vi "Build Control Type.vi"(8 "error in (no error)":errorcluster, 11 "Button Builder.lvclass":refnum<class "Button_Builder.lvclass">) -> (0 "error out":errorcluster, 2 "GUI Control":refnum<class "GUI Control.lvclass">, 3 "Button Builder.lvclass out":refnum<class "Button_Builder.lvclass">)   [LabVIEW 2015, in "Button_Builder.lvclass"]
uses:
  Button_Builder.lvclass
  GUI Controls/GUI Control/GUI Control.lvclass
  Panel Control/Panel Data/Type Definition/Panel Control Maker State Variable.ctl
  GUI Controls/Button_UI/Button_UI.lvclass
  Panel Control_Ref/Panel Controller.lvclass
  <vilib>/Utility/error.llb/Error Cluster From Error Code.vi
  <vilib>/ErrorRing/Error Ring.xnode
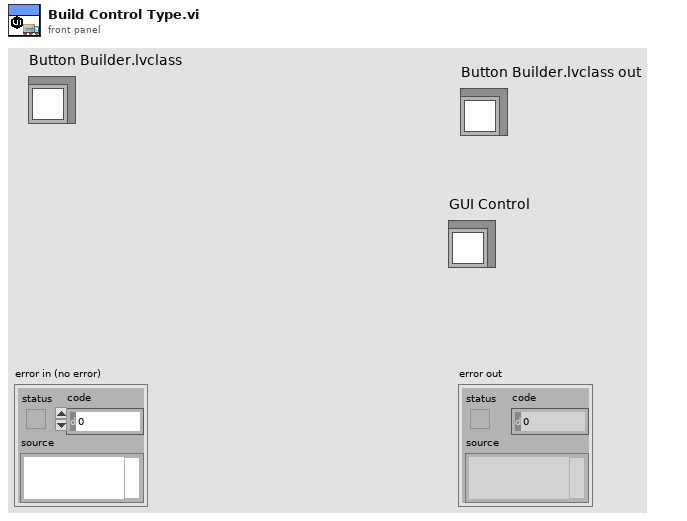
[diagram p1: front panel]
types:
  T1 = typedef "Panel Controller.lvclass/Panel Control Maker State Variable.ctl" = enum16{"Panel On", "Working", "Panel Off", "Ending"}
  T2 = enum32{"Invalid", "Standard", "Closed", "Hidden", "Minimized", "Maximized"}
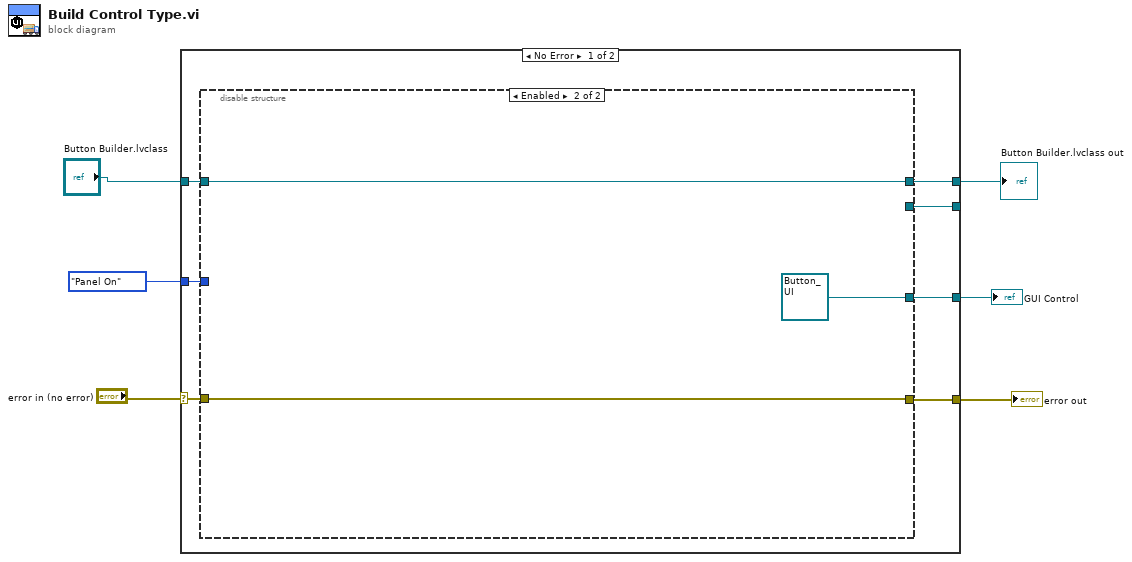
[diagram p0: block diagram]
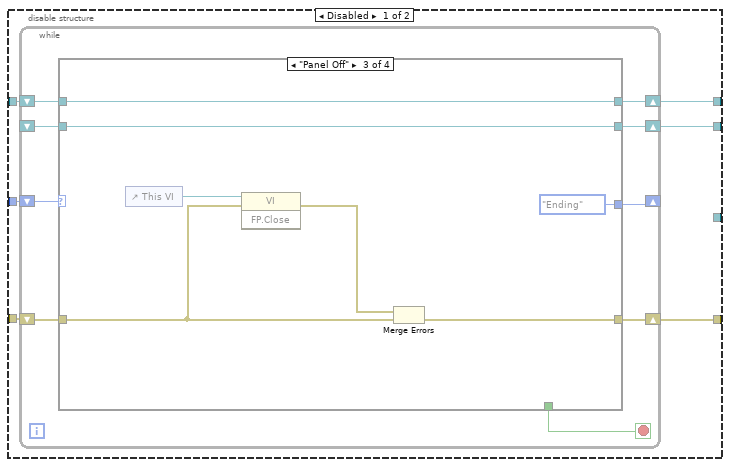
[diagram p2: hidden frame]
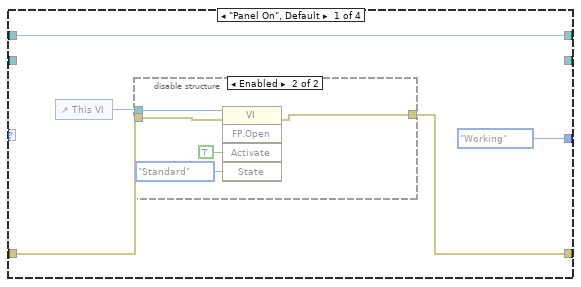
[diagram p3: hidden frame]
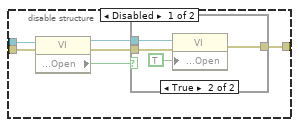
[diagram p4: hidden frame]
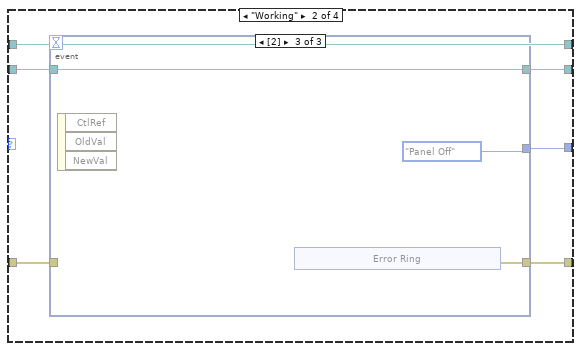
[diagram p6: hidden frame]
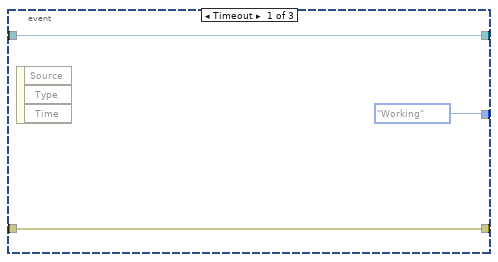
[diagram p7: hidden frame]
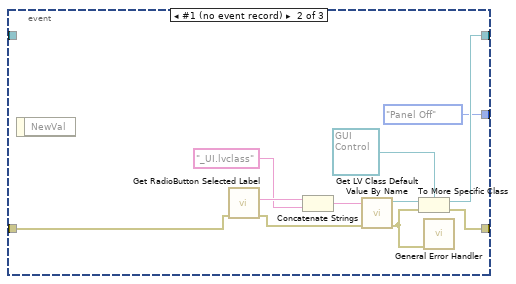
[diagram p8: hidden frame]
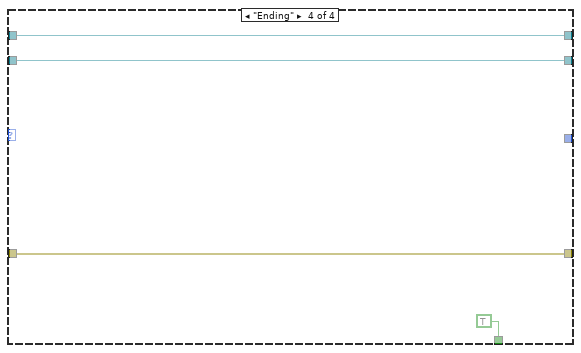
[diagram p9: hidden frame]
diagram:
  n1 = case shown="No Error" "error in (no error)" {
    selector: "error in (no error)" -> [w12 w94]
    tunnel: Panel_Control_Maker_State_Variable."Panel On" -> [w13 _]
    tunnel: [w11 w94] -> w4
    tunnel: [w10 _] -> _
    tunnel: "Button Builder.lvclass" -> [w9 w93]
    tunnel: [w8 w93] -> w1
    tunnel: [w7 _] -> w3
    frame No Error {
      n2 = disable-structure shown="Enabled" {
        disable-tunnel: w13 -> [w19 _]
        disable-tunnel: w12 -> [w18 w90]
        disable-tunnel: [w17 w90] -> w11
        disable-tunnel: [w16 _] -> w10
        disable-tunnel: w9 -> [w15 w92]
        disable-tunnel: [w14 w92] -> w8
        disable-tunnel: [_ refnum<class "Button_UI.lvclass"> refnum ("Button_UI")] -> w7
        frame Disabled {
          n3 = while {
            shift-right: [w25] -> _
            shift-left: w19 -> [w28]
            shift-right: [w26] -> w17
            shift-left: w18 -> [w27]
            shift-right: [w24] -> w16
            shift-left: _ -> [w23]
            shift-right: [w20] -> w14
            shift-left: w15 -> [w21]
            stop <- w22 stop-if-true
            n4 = case shown="\"Panel Off\"" w28 {
              tunnel: w27 -> [w32 w51 w81 w88]
              tunnel: [w31 w52 w83 w88] -> w26
              tunnel: [Panel_Control_Maker_State_Variable."Working" w53 Panel_Control_Maker_State_Variable."Ending" _] -> w25
              tunnel: [_ w55 w85 w86] -> w24
              tunnel: w23 -> [_ w54 w85 w86]
              tunnel: [_ _ _ TRUE] -> w22
              tunnel: w21 -> [w29 w50 w79 w87]
              tunnel: [w29 w50 w79 w87] -> w20
              frame "Panel On", Default {
                n5 = control-ref of="This VI"() -> (w33:refnum<vi>)
                n6 = disable-structure shown="Enabled" {
                  disable-tunnel: w33 -> [w39 w49]
                  disable-tunnel: w32 -> [w38 w48]
                  disable-tunnel: [w34 w47] -> w31
                  frame Disabled {
                    n7 = property class="VI"(reference=w39, error in=w38) -> (reference out=w35:refnum<vi>, error out=w36:errorcluster, "Front Panel.Open"=w37:bool)
                    n8 = case shown="True" w37 {
                      tunnel: w36 -> [w40 w43]
                      tunnel: w35 -> [_ w44]
                      tunnel: [w40 w41] -> w34
                      frame False {
                      }
                      frame True {
                        n9 = property class="VI"(reference=w44, error in=w43, "Front Panel.Open"=TRUE ("Front Panel Window:Open")) -> (error out=w41:errorcluster)  [unwired: 1 out]
                      }
                    }
                  }
                  frame Enabled {
                    n10 = invoke class="VI" method="FP.Open"(reference=w49, error in=w48, "Activate"=TRUE ("Activate?"), "State"=T2."Standard") -> (error out=w47:errorcluster)  [unwired: 1 in, 4 out]
                  }
                }
              }
              frame "Working" {
                n11 = event shown="[2]" {
                  selector: _ -> [_ _ _]
                  dyn-events: _ -> [_ _ _]
                  timeout: _ -> [_ _ _]
                  tunnel: [w56 w64 w73] -> w52
                  tunnel: [w57 w63 w72] -> w55
                  tunnel: w54 -> [w57 _ w72]
                  tunnel: [Panel_Control_Maker_State_Variable."Working" Panel_Control_Maker_State_Variable."Panel Off" Panel_Control_Maker_State_Variable."Panel Off"] -> w53
                  tunnel: w51 -> [w56 w61 _]
                  event Timeout {
                    n12 = event-data() -> ()  [unwired: 1 in, 3 out]
                  }
                  event #1 (no event record) {
                    n13 = event-data() -> ()  [unwired: 1 in, 1 out]
                    n14 = call "Get RadioButton Selected Label.vi"("error in (no error)"=w61) -> ("error out"=w60:errorcluster, "Label.Text"=w69:string, "Radio Buttons"=w70:refnum<vi>)  [unwired: 7 in, 1 out]
                    n15 = Concatenate Strings(w69, "_UI.lvclass" ("string")) -> (w67:string)
                    n16 = call <vilib>:"Get LV Class Default Value By Name.vi"("error in (no error)"=w60, "class name"=w67) -> ("error out"=w59:errorcluster, "object"=w66:refnum<class>)  [unwired: 8 in]
                    n17 = To More Specific Class(target class=refnum<class "GUI Control.lvclass"> refnum ("GUI Control"), reference=w66, error in=w59) -> (specific class reference=w63:refnum<class "GUI Control.lvclass">, error out=w64:errorcluster)
                    n18 = call <vilib>:"General Error Handler.vi"("error in (no error)"=w59) -> ()  [unwired: 10 in, 5 out]
                  }
                  event #2 (no event record) {
                    n19 = event-data() -> ()  [unwired: 1 in, 3 out]
                    n20 = xnode "Error Ring"() -> ("error out"=w73:errorcluster)
                  }
                }
              }
              frame "Panel Off" {
                n21 = control-ref of="This VI"() -> (w82:refnum<vi>)
                n22 = invoke class="VI" method="FP.Close"(reference=w82, error in=w81) -> (error out=w80:errorcluster)  [unwired: 1 in, 2 out]
                n23 = Merge Errors(w80, w81) -> (w83:errorcluster)
              }
              frame "Ending" {
              }
            }
          }
        }
        frame Enabled {
        }
      }
    }
    frame Error {
    }
  }
  "error out" <- w4
  "GUI Control" <- w3
  "Button Builder.lvclass out" <- w1
